vi "GetCoordinates.vi"(7 "# row":i32, 8 "# col":i32, 9 "Row":i32, 10 "Col":i32) -> (1 "Arraytest":i32[][](array[numeric]), 3 "ArrayNeighbours":i32[][](array[numeric]))   [LabVIEW 2013]
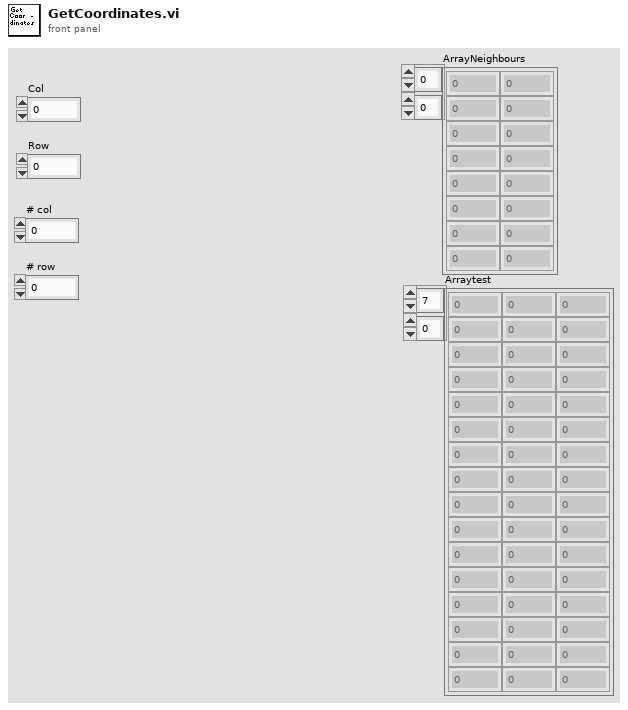
[diagram p1: front panel]
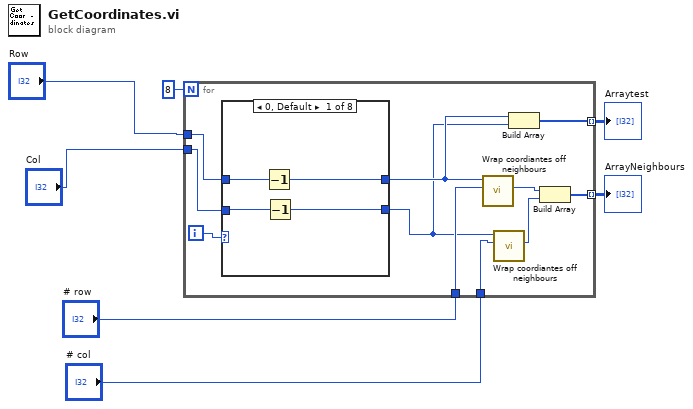
[diagram p0: block diagram]
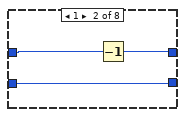
[diagram p2: hidden frame]
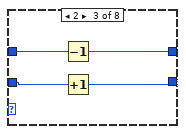
[diagram p3: hidden frame]
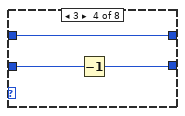
[diagram p4: hidden frame]
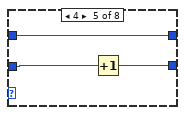
[diagram p5: hidden frame]
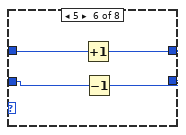
[diagram p6: hidden frame]
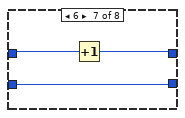
[diagram p7: hidden frame]
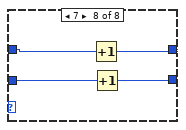
[diagram p8: hidden frame]
diagram:
  n1 = for {
    N: 8 -> [_]
    tunnel: "Col" -> [w16]
    tunnel: "Row" -> [w17]
    tunnel: "# row" -> [w15]
    tunnel: "# col" -> [w14]
    tunnel: [w12] -> w2 mode=indexing
    tunnel: [w9] -> w1 mode=indexing
    i -> [w18]
    n2 = case shown="0, Default" w18 {
      tunnel: w17 -> [w22 w24 w29 w32 w35 w39 w41 w46]
      tunnel: w16 -> [w21 w25 w27 w31 w34 w37 w42 w44]
      tunnel: [w20 w23 w28 w32 w35 w38 w40 w45] -> w11
      tunnel: [w19 w25 w26 w30 w33 w36 w42 w43] -> w10
      frame 0, Default {
        n3 = Decrement(x=w22) -> (x-1=w20:i32)
        n4 = Decrement(x=w21) -> (x-1=w19:i32)
      }
      frame 1 {
        n5 = Decrement(x=w24) -> (x-1=w23:i32)
      }
      frame 2 {
        n6 = Decrement(x=w29) -> (x-1=w28:i32)
        n7 = Increment(x=w27) -> (x+1=w26:i32)
      }
      frame 3 {
        n8 = Decrement(x=w31) -> (x-1=w30:i32)
      }
      frame 4 {
        n9 = Increment(x=w34) -> (x+1=w33:i32)
      }
      frame 5 {
        n10 = Increment(x=w39) -> (x+1=w38:i32)
        n11 = Decrement(x=w37) -> (x-1=w36:i32)
      }
      frame 6 {
        n12 = Increment(x=w41) -> (x+1=w40:i32)
      }
      frame 7 {
        n13 = Increment(x=w46) -> (x+1=w45:i32)
        n14 = Increment(x=w44) -> (x+1=w43:i32)
      }
    }
    n15 = call "Wrap coordiantes off neighbours.vi"("Length"=w15, "Index"=w11) -> ("Translated index"=w8:i32)  [unwired: 9 in]
    n16 = call "Wrap coordiantes off neighbours.vi"("Length"=w14, "Index"=w10) -> ("Translated index"=w13:i32)  [unwired: 9 in]
    n17 = Build Array(w11, w10) -> (w9:i32[])
    n18 = Build Array(w8, w13) -> (w12:i32[])
  }
  "ArrayNeighbours" <- w2
  "Arraytest" <- w1
